vi "toTimestamp.vi"(7 "Use TAI Offset?":bool=TRUE, 9 "Fractional Second":dbl format="%#.6f", 10 "GPS Time (s)":i64, 11 "Epoch (GPS)":refnum<class "Epoch.GPS.lvclass">) -> (1 "Not a Timestamp?":bool, 2 "Timestamp":timestamp, 3 "Epoch out":refnum<class "Epoch.GPS.lvclass">)   [LabVIEW 2013, in "Epoch.GPS.lvclass"]
uses:
  Epoch.GPS.lvclass
  epoch/Epoch.lvclass
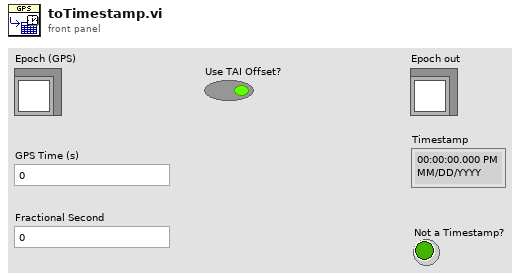
[diagram p1: front panel]
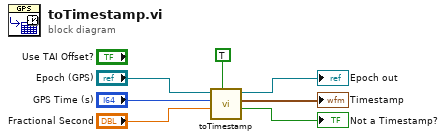
[diagram p0: block diagram]
diagram:
  n1 = call-parent "toTimestamp.vi"("Use TAI Offset?"=TRUE, "Fractional Second"="Fractional Second", "Epoch Time (s)"="GPS Time (s)", "Epoch (Local)"="Epoch (GPS)") -> ("Not a Timestamp?"=→"Not a Timestamp?":bool, "Timestamp"=→"Timestamp":timestamp, "Epoch (out)"=→"Epoch out":refnum<class "Epoch.GPS.lvclass">)  [unwired: 5 in]
